vi "onGenerateNewInboundChannel.vi"(8 "error in (no error)":errorcluster, 11 "Connection in":refnum<class "Connection.lvclass">) -> (0 "error out":errorcluster, 3 "Connection out":refnum<class "Connection.lvclass">)   [LabVIEW 2013, in "Connection_GOSPL.lvlib" / "Connection.lvclass"]
uses:
  Connection.lvclass
  Connection.lvclass/Connection.ctl
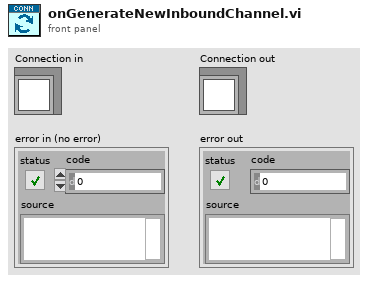
[diagram p1: front panel]
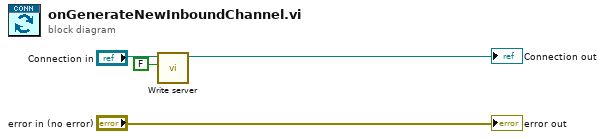
[diagram p0: block diagram]
diagram:
  n1 = call "Write server.vi"("server"=FALSE, "Connection in"="Connection in") -> ("Connection out"=→"Connection out":refnum<class "Connection.lvclass">)  [unwired: 9 in]
  "error out" <- "error in (no error)"
